vi "AndorInit.vi"(0 "TargetTemp":i32, 5 "error in":errorcluster, 7 "CoolerONRef":refnum<vi>, 8 "GetStatusRef":refnum<vi>, 9 "CurrentTempRef":refnum<vi>) -> (10 "GetStatus":T2, 11 "CurrentTemp":i32, 13 "CoolerON":T1, 14 "DevInit":bool, 15 "DevSize":cluster{"xpixels":i32, "ypixels":i32}, 16 "HardWVersion":T5, 17 "SoftWVersion":T4, 18 "Speeds":T3, 19 "error out":errorcluster)   [LabVIEW 2014]
uses:
  <userlib>/atmcd64d.llb/HSSpeed_type typedef.ctl
  <userlib>/atmcd64d.llb/Error Code Enum typedef.ctl
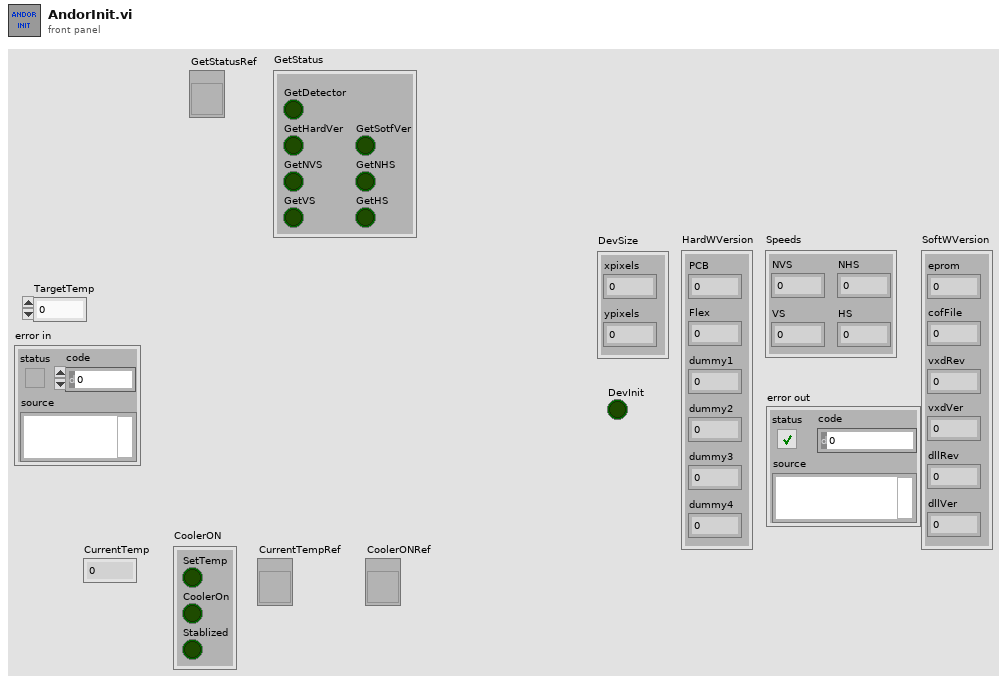
[diagram p1: front panel]
types:
  T1 = cluster{"SetTemp":bool, "CoolerOn":bool, "Stablized":bool}
  T2 = cluster{"GetDetector":bool, "GetHardVer":bool, "GetNVS":bool, "GetVS":bool, "GetSotfVer":bool, "GetNHS":bool, "GetHS":bool}
  T3 = cluster{"NVS":i32, "VS":i32, "NHS":dbl, "HS":i32}
  T4 = cluster{"eprom":u32, "cofFile":u32, "vxdRev":u32, "vxdVer":u32, "dllRev":u32, "dllVer":u32}
  T5 = cluster{"PCB":u32, "Flex":u32, "dummy1":u32, "dummy2":u32, "dummy3":u32, "dummy4":u32}
  T6 = typedef "HSSpeed_type typedef.ctl" = enum16{"EM Amp", "Conventional Amp"}
  T7 = typedef "Error Code Enum typedef.ctl" = enum32{"N/A (0)", "DRV_ERROR_CODES", "DRV_SUCCESS", "DRV_VXDNOTINSTALLED", "DRV_ERROR_SCAN", "DRV_ERROR_CHECK_SUM", "DRV_ERROR_FILELOAD", "DRV_UNKNOWN_FUNC", "DRV_ERROR_VXD_INIT", "DRV_ERROR_ADDRESS", "DRV_ERROR_PAGELOCK", "DRV_ERROR_PAGEUNLOCK", "DRV_ERROR_BOARDTEST", "DRV_ERROR_ACK", "DRV_ERROR_UP_FIFO", "DRV_ERROR_PATTERN", "N/A (16)", "DRV_ACQUISITION_ERRORS", "DRV_ACQ_BUFFER", "DRV_ACQ_DOWNFIFO_FULL", "DRV_PROC_UNKONWN_INSTRUCTION", "DRV_ILLEGAL_OP_CODE", "DRV_KINETIC_TIME_NOT_MET", "DRV_ACCUM_TIME_NOT_MET", "DRV_NO_NEW_DATA", "N/A (25)", "DRV_SPOOLERROR", "N/A (27)", "N/A (28)", "N/A (29)", "N/A (30)", "N/A (31)", "N/A (32)", "DRV_TEMPERATURE_CODES", "DRV_TEMPERATURE_OFF", "DRV_TEMPERATURE_NOT_STABILIZED", "DRV_TEMPERATURE_STABILIZED", "DRV_TEMPERATURE_NOT_REACHED", "DRV_TEMPERATURE_OUT_RANGE", "DRV_TEMPERATURE_NOT_SUPPORTED", "DRV_TEMPERATURE_DRIFT", "N/A (41)", "N/A (42)", "N/A (43)", "N/A (44)", "N/A (45)", "N/A (46)", "N/A (47)", "N/A (48)", "DRV_GENERAL_ERRORS", "DRV_INVALID_AUX", "DRV_COF_NOTLOADED", "DRV_FPGAPROG", "DRV_FLEXERROR", "DRV_GPIBERROR", "N/A (55)", "N/A (56)", "N/A (57)", "N/A (58)", "N/A (59)", "N/A (60)", "N/A (61)", "N/A (62)", "N/A (63)", "DRV_DATATYPE", "DRV_DRIVER_ERRORS", "DRV_P1INVALID", "DRV_P2INVALID", "DRV_P3INVALID", "DRV_P4INVALID", "DRV_INIERROR", "DRV_COFERROR", "DRV_ACQUIRING", "DRV_IDLE", "DRV_TEMPCYCLE", "DRV_NOT_INITIALIZED", "DRV_P5INVALID", "DRV_P6INVALID", "DRV_INVALID_MODE", "DRV_INVALID_FILTER", "DRV_I2CERRORS", "DRV_I2CDEVNOTFOUND", "DRV_I2CTIMEOUT", "DRV_P7INVALID", "N/A (84)", "N/A (85)", "N/A (86)", "N/A (87)", "N/A (88)", "N/A (89)", "DRV_IOCERROR", "DRV_VRMVERSIONERROR"}
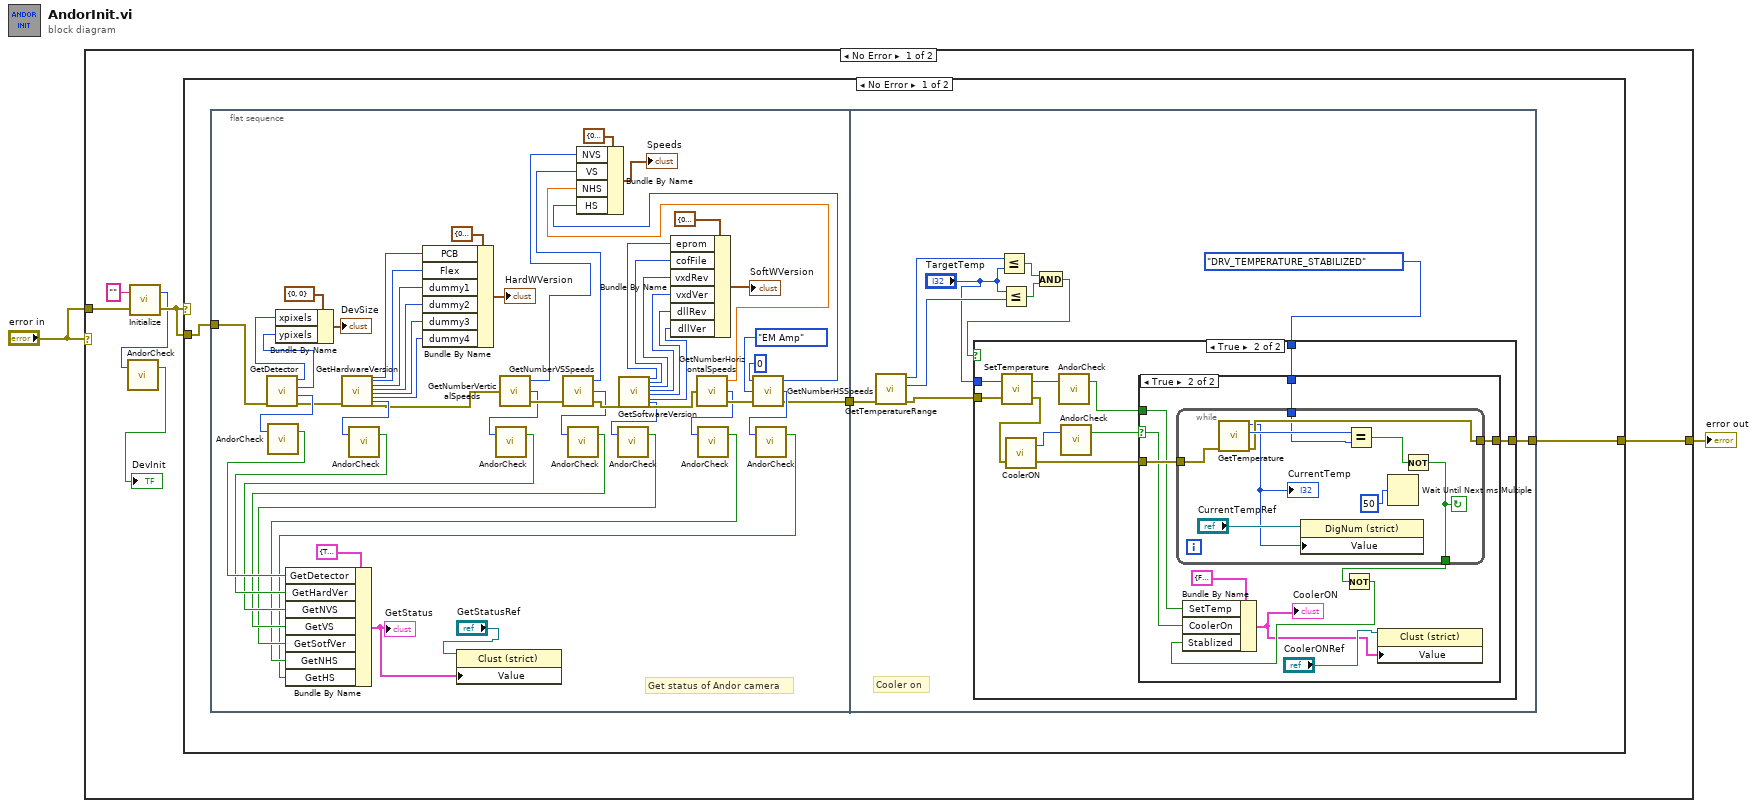
[diagram p0: block diagram]
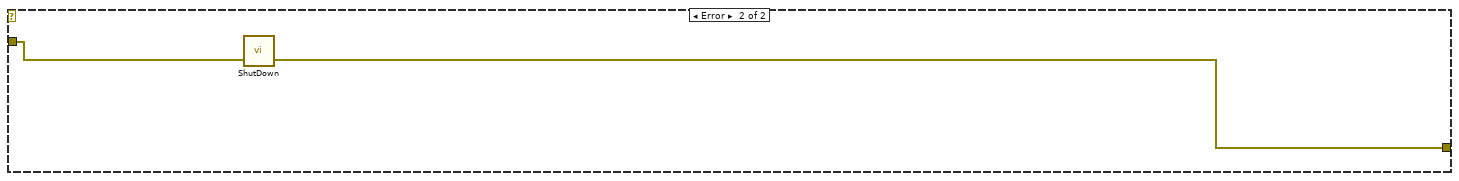
[diagram p4: hidden frame]
diagram:
  n1 = case shown="No Error" "error in" {
    tunnel: "error in" -> [w8 w108]
    tunnel: [w3 w108] -> w1
    frame No Error {
      n2 = call <userlib>:"Initialize.vi"("error in (no error)"=w8, "directory (\"\")"="" ("directory (\"\")")) -> ("error out"=w7:errorcluster, "DLL error code"=w6:u32)
      n3 = call "AndorCheck.vi"("Input"=w6) -> ("Status"=→"DevInit":bool)  [unwired: 1 in, 1 out]
      n4 = case shown="No Error" w7 {
        tunnel: w7 -> [w11 w107]
        tunnel: [w9 w106] -> w3
        frame No Error {
          n5 = flat-sequence {
            tunnel: w11 -> [w64]
            tunnel: [w14] -> w10
            tunnel: w10 -> [w74]
            tunnel: [w66] -> w9
            frame #0 {
              # "Get status of Andor camera"
              n6 = call <userlib>:"GetDetector.vi"("error in (no error)"=w64) -> ("error out"=w58:errorcluster, "DLL error code"=w59:u32, "ypixels"=w61:i32, "xpixels"=w62:i32)  [unwired: 3 in]
              n7 = call "AndorCheck.vi"("Input"=w59) -> ("Status"=w21:bool)  [unwired: 1 in, 1 out]
              n8 = Bundle By Name(cluster=cluster{"xpixels":i32, "ypixels":i32} {"xpixels"=0, "ypixels"=0} ("DevSize"), "xpixels"=w62, "ypixels"=w61) -> (→"DevSize":cluster{"xpixels":i32, "ypixels":i32})
              n9 = call <userlib>:"GetHardwareVersion.vi"("error in (no error)"=w58) -> ("PCB"=w55:u32, "Flex"=w54:u32, "dummy1"=w53:u32, "dummy2"=w52:u32, "dummy3"=w51:u32, "dummy4"=w50:u32, "DLL error code"=w49:u32, "error out"=w48:errorcluster)  [unwired: 19 in]
              n10 = call "AndorCheck.vi"("Input"=w49) -> ("Status"=w20:bool)  [unwired: 1 in, 1 out]
              n11 = Bundle By Name(cluster=T5 {"PCB"=0, "Flex"=0, "dummy1"=0, "dummy2"=0, "dummy3"=0, "dummy4"=0} ("HardWVersion"), "PCB"=w55, "Flex"=w54, "dummy1"=w53, "dummy2"=w52, "dummy3"=w51, "dummy4"=w50) -> (→"HardWVersion":T5)
              n12 = call <userlib>:"GetNumberVerticalSpeeds.vi"("error in (no error)"=w48) -> ("number"=w29:i32, "Dll Error Code"=w36:u32, "error out"=w47:errorcluster)
              n13 = call "AndorCheck.vi"("Input"=w36) -> ("Status"=w19:bool)  [unwired: 1 in, 1 out]
              n14 = call <userlib>:"GetNumberVSSpeeds.vi"("error in (no error)"=w47) -> ("error out"=w45:errorcluster, "DLL error code"=w35:u32, "number"=w28:i32)  [unwired: 2 in]
              n15 = call "AndorCheck.vi"("Input"=w35) -> ("Status"=w18:bool)  [unwired: 1 in, 1 out]
              n16 = call <userlib>:"GetSoftwareVersion.vi"("error in (no error)"=w45) -> ("eprom"=w41:u32, "cofFile"=w40:u32, "vxdRev"=w39:u32, "vxdVer"=w38:u32, "dllRev"=w37:u32, "dllVer"=w23:u32, "DLL error code"=w34:u32, "error out"=w44:errorcluster)  [unwired: 19 in]
              n17 = call "AndorCheck.vi"("Input"=w34) -> ("Status"=w17:bool)  [unwired: 1 in, 1 out]
              n18 = Bundle By Name(cluster=T4 {"eprom"=0, "cofFile"=0, "vxdRev"=0, "vxdVer"=0, "dllRev"=0, "dllVer"=0} ("SoftWVersion"), "eprom"=w41, "cofFile"=w40, "vxdRev"=w39, "vxdVer"=w38, "dllRev"=w37, "dllVer"=w23) -> (→"SoftWVersion":T4)
              n19 = call <userlib>:"GetNumberHorizontalSpeeds.vi"("error in (no error)"=w44) -> ("number"=w26:dbl, "Dll Error Code"=w33:u32, "error out"=w46:errorcluster)
              n20 = call "AndorCheck.vi"("Input"=w33) -> ("Status"=w16:bool)  [unwired: 1 in, 1 out]
              n21 = call <userlib>:"GetNumberHSSpeeds.vi"("error in (no error)"=w46, "type"=HSSpeed_type_typedef."EM Amp", "channel"=0) -> ("error out"=w14:errorcluster, "DLL error code"=w32:u32, "number"=w27:i32)
              n22 = Bundle By Name(cluster=T3 {"NVS"=0, "VS"=0, "NHS"=0.0, "HS"=0} ("Speeds"), "NVS"=w29, "VS"=w28, "NHS"=w26, "HS"=w27) -> (→"Speeds":T3)
              n23 = call "AndorCheck.vi"("Input"=w32) -> ("Status"=w15:bool)  [unwired: 1 in, 1 out]
              n24 = Bundle By Name(cluster=T2 {"GetDetector"=TRUE, "GetHardVer"=TRUE, "GetNVS"=TRUE, "GetVS"=TRUE, "GetSotfVer"=TRUE, "GetNHS"=TRUE, "GetHS"=TRUE} ("GetStatus"), "GetDetector"=w21, "GetHardVer"=w20, "GetNVS"=w19, "GetVS"=w18, "GetSotfVer"=w17, "GetNHS"=w16, "GetHS"=w15) -> (w12:T2)
              "GetStatus" <- w12
              n25 = property class="Clust (strict)"(reference="GetStatusRef", "Value"=w12) -> ()  [unwired: 1 in, 2 out]
            }
            frame #1 {
              # "Cooler on"
              n26 = call <userlib>:"GetTemperatureRange.vi"("error in (no error)"=w74) -> ("error out"=w69:errorcluster, "maxTemp"=w72:i32, "minTemp"=w73:i32)  [unwired: 3 in, 1 out]
              n27 = Less Or Equal?(x=w73, y="TargetTemp") -> (x <= y?=w70:bool)
              n28 = Less Or Equal?(x="TargetTemp", y=w72) -> (x <= y?=w71:bool)
              n29 = And(x=w70, y=w71) -> (x .and. y?=w68:bool)
              n30 = case shown="True" w68 {
                tunnel: w69 -> [w75 w85]
                tunnel: "TargetTemp" -> [_ w84]
                tunnel: [w75 w79] -> w66
                tunnel: Error_Code_Enum_typedef."DRV_TEMPERATURE_STABILIZED" ("y") -> [_ w76]
                frame False {
                }
                frame True {
                  n31 = call <userlib>:"SetTemperature.vi"("error in (no error)"=w85, "temperature"=w84) -> ("error out"=w83:errorcluster, "DLL error code"=w82:u32)
                  n32 = call <userlib>:"CoolerON.vi"("error in (no error)"=w83) -> ("error out"=w80:errorcluster, "DLL error code"=w81:u32)  [unwired: 1 in]
                  n33 = call "AndorCheck.vi"("Input"=w82) -> ("Status"=w77:bool)  [unwired: 1 in, 1 out]
                  n34 = call "AndorCheck.vi"("Input"=w81) -> ("Status"=w78:bool)  [unwired: 1 in, 1 out]
                  n35 = case shown="True" w78 {
                    selector: w78 -> [_ w89]
                    tunnel: w80 -> [w86 w96]
                    tunnel: [w86 w95] -> w79
                    tunnel: w77 -> [_ w90]
                    tunnel: w76 -> [_ w87]
                    frame False {
                    }
                    frame True {
                      n36 = while {
                        tunnel: w96 -> [w105]
                        tunnel: [w100] -> w95
                        tunnel: [w101] -> w94
                        tunnel: w87 -> [w97]
                        stop <- w101 continue-if-true
                        n37 = call <userlib>:"GetTemperature.vi"("error in (no error)"=w105) -> ("error out"=w100:errorcluster, "status"=w104:T7, "temperature"=w98:i32)  [unwired: 3 in, 1 out]
                        "CurrentTemp" <- w98
                        n38 = property class="DigNum (strict)"(reference="CurrentTempRef", "Value"=w98) -> ()  [unwired: 1 in, 2 out]
                        n39 = Equal?(x=w104, y=w97) -> (x = y?=w103:bool)
                        n40 = Wait Until Next ms Multiple(millisecond multiple=u32 50) -> ()  [unwired: 1 out]
                        n41 = Not(x=w103) -> (.not. x?=w101:bool)
                      }
                      n42 = Not(x=w94) -> (.not. x?=w91:bool)
                      n43 = Bundle By Name(cluster=T1 {"SetTemp"=FALSE, "CoolerOn"=FALSE, "Stablized"=FALSE} ("CoolerON"), "SetTemp"=w90, "CoolerOn"=w89, "Stablized"=w91) -> (w88:T1)
                      "CoolerON" <- w88
                      n44 = property class="Clust (strict)"(reference="CoolerONRef", "Value"=w88) -> ()  [unwired: 1 in, 2 out]
                    }
                  }
                }
              }
            }
          }
        }
        frame Error {
          n45 = call <userlib>:"ShutDown.vi"("error in (no error)"=w107) -> ("error out"=w106:errorcluster)  [unwired: 1 in, 1 out]
        }
      }
    }
    frame Error {
    }
  }
  "error out" <- w1
